vi "Create Folder at Location.vi"(5 "Override existing (F)":bool, 7 "Use Relative (F)":bool, 8 "Error In":errorcluster, 10 "Path":string) -> (0 "Error Out":errorcluster, 1 "Already Exists ?":bool, 2 "Full path out":path)   [LabVIEW 2019, in "gRPC Scripting Tools.lvlib"]
uses:
  gRPC Scripting Tools.lvlib
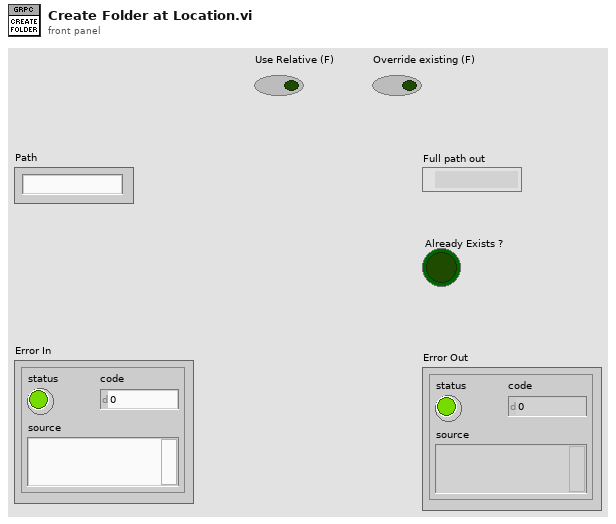
[diagram p1: front panel]
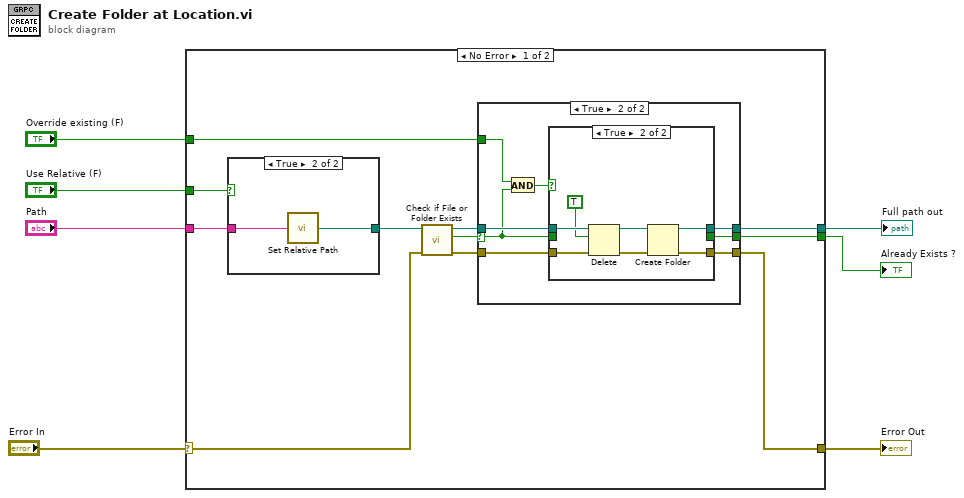
[diagram p0: block diagram]
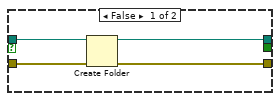
[diagram p2: hidden frame]
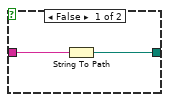
[diagram p4: hidden frame]
diagram:
  n1 = case shown="No Error" "Error In" {
    selector: "Error In" -> [w15 w45]
    tunnel: "Path" -> [w17 _]
    tunnel: "Use Relative (F)" -> [w18 _]
    tunnel: "Override existing (F)" -> [w11 _]
    tunnel: [w10 w45] -> w3
    tunnel: [w9 _] -> w2
    tunnel: [w8 _] -> w1
    frame No Error {
      n2 = case shown="True" w18 {
        tunnel: w17 -> [w42 w44]
        tunnel: [w41 w43] -> w16
        frame False {
          n3 = String To Path(string=w42) -> (path=w41:path)
        }
        frame True {
          n4 = call "Set Relative Path.vi"("Application Relative Path"=w44) -> ("Full Path"=w43:path)
        }
      }
      n5 = call <vilib>:"Check if File or Folder Exists.vi"("error in (no error)"=w15, "path"=w16) -> ("error out"=w12:errorcluster, "file or folder exists?"=w14:bool, "dup path"=w13:path)  [unwired: 7 in]
      n6 = case shown="True" w14 {
        selector: w14 -> [_ w24]
        tunnel: w13 -> [w21 w30]
        tunnel: w12 -> [w22 w27]
        tunnel: w11 -> [_ w29]
        tunnel: [w19 w26] -> w9
        tunnel: [w20 w25] -> w10
        tunnel: [_ w23] -> w8
        frame False {
          n7 = Create Folder(path (use dialog)=w21, error in=w22) -> (created path=w19:path, error out=w20:errorcluster)  [unwired: 1 in, 1 out]
        }
        frame True {
          n8 = And(x=w29, y=w24) -> (x .and. y?=w28:bool)
          n9 = case shown="True" w28 {
            tunnel: w30 -> [w33 w40]
            tunnel: w27 -> [w32 w38]
            tunnel: [w32 w34] -> w25
            tunnel: [w33 w35] -> w26
            tunnel: w24 -> [w31 _]
            tunnel: [w31 _] -> w23
            frame False {
            }
            frame True {
              n10 = Delete(path (use dialog)=w40, entire hierarchy (F)=TRUE, error in=w38) -> (deleted path=w36:path, error out=w37:errorcluster)  [unwired: 2 in, 1 out]
              n11 = Create Folder(path (use dialog)=w36, error in=w37) -> (created path=w35:path, error out=w34:errorcluster)  [unwired: 1 in, 1 out]
            }
          }
        }
      }
    }
    frame Error {
    }
  }
  "Error Out" <- w3
  "Full path out" <- w2
  "Already Exists ?" <- w1
